vi "Initialize QA Session.vi"(0 "resonator labels":string[](array[string]), 1 "Oximetry Mode?":bool, 5 "Sample Selection":string[](array[string])=["None v1", "T10-1 v1", "T10-10 v1", "T10-11 v1", "T10-12 v1", "T10-13 v1", "T10-14 v1", "T10-15 v1", "T10-16 v1", "T10-17 v1", "T10-2 v1", "T10-3 v1", "T10-4 v1", "T10-5 v1", "T10-6 v1", "T10-7 v1", "T10-8 v1", "T10-9 v1", "T1-10 v1", "T1-11 v1", "T11-1 v1", "T11-10 v1", "T11-11 v1", "T11-12 v1", "T11-13 v1", "T11-14 v1", "T11-15 v1", "T11-16 v1", "T11-17 v1", "T11-18 v1", "T11-19 v1", "T1-12 v1", "T11-2 v1", "T11-20 v1", "T11-21 v1", "T11-22 v1", "T11-23 v1", "T11-24 v1", "T11-25 v1", "T11-26 v1", "T11-27 v1", "T11-28 v1", "T11-29 v1", "T1-13 v1", "T11-3 v1", "T11-30 v1", "T11-31 v1", "T11-32 v1", "T11-33 v1", "T11-34 v1", "T11-35 v1", "T11-36 v1", "T11-37 v1", "T11-38 v1", "T11-39 v1", "T1-14 v1", "T11-4 v1", "T11-40 v1", "T11-41 v1", "T11-42 v1", "T1-15 v1", "T11-5 v1", "T1-16 v1", "T11-6 v1", "T1-17 v1", "T11-7 v1", "T1-18 v1", "T11-8 v1", "T1-19 v1", "T11-9 v1", "T1-2 v1", "T1-2 v2", "T1-2 v3", "T1-20 v1", "T1-21 v1", "T12-1 v1", "T12-10 v1", "T12-11 v1", "T12-12 v1", "T12-13 v1", "T12-14 v1", "T12-15 v1", "T12-16 v1", "T12-17 v1", "T12-18 v1", "T12-19 v1", "T1-22 v1", "T12-2 v1", "T1-23 v1", "T12-3 v1", "T1-24 v1", "T12-4 v1", "T1-25 v1", "T12-5 v1", "T1-26 v1", "T12-6 v1", "T1-27 v1", "T12-7 v1", "T1-28 v1", "T12-8 v1", "T1-29 v1", "T12-9 v1", "T1-3 v1", "T13-10 v1", "T13-11 v1", "T13-12 v1", "T13-13 v1", "T13-2 v1", "T13-3 v1", "T13-4 v1", "T13-5 v1", "T13-6 v1", "T13-7 v1", "T13-8 v1", "T13-9 v1", "T1-4 v1", "T14-1 v1", "T14-10 v1", "T14-11 v1", "T14-12 v1", "T14-13 v1", "T14-14 v1", "T14-15 v1", "T14-16 v1", "T14-17 v1", "T14-2 v1", "T14-3 v1", "T14-4 v1", "T14-5 v1", "T14-6 v1", "T14-7 v1", "T14-8 v1", "T14-9 v1", "T1-5 v1", "T1-5 v2", "T15-1 v1", "T15-10 v1", "T15-11 v1", "T15-2 v1", "T15-3 v1", "T15-4 v1", "T15-5 v1", "T15-6 v1", "T15-7 v1", "T15-8 v1", "T15-9 v1", "T1-6 v1", "T1-6 v2", "T16-1 v1", "T16-10 v1", "T16-11 v1", "T16-12 v1", "T16-13 v1", "T16-14 v1", "T16-15 v1", "T16-16 v1", "T16-17 v1", "T16-18 v1", "T16-19 v1", "T16-2 v1", "T16-20 v1", "T16-21 v1", "T16-22 v1", "T16-23 v1", "T16-24 v1", "T16-25 v1", "T16-3 v1", "T16-4 v1", "T16-5 v1", "T16-6 v1", "T16-7 v1", "T16-8 v1", "T16-9 v1", "T1-7 v1", "T17-1 v1", "T17-10 v1", "T17-11 v1", "T17-12 v1", "T17-13 v1", "T17-14 v1", "T17-15 v1", "T17-16 v1", "T17-17 v1", "T17-2 v1", "T17-3 v1", "T17-4 v1", "T17-5 v1", "T17-6 v1", "T17-7 v1", "T17-8 v1", "T17-9 v1", "T1-8 v1", "T18-1 v1", "T18-2 v1", "T18-3 v1", "T18-4 v1", "T18-5 v1", "T18-6 v1", "T18-7 v1", "T18-8 v1", "T18-9 v1", "T1-9 v1", "T19-1 v1", "T19-10 v1", "T19-11 v1", "T19-12 v1", "T19-13 v1", "T19-14 v1", "T19-15 v1", "T19-16 v1", "T19-17 v1", "T19-18 v1", "T19-19 v1", "T19-2 v1", "T19-3 v1", "T19-4 v1", "T19-5 v1", "T19-6 v1", "T19-7 v1", "T19-8 v1", "T19-9 v1", "T20-1 v1", "T20-10 v1", "T20-11 v1", "T20-12 v1", "T20-13 v1", "T20-14 v1", "T20-2 v1", "T20-3 v1", "T20-4 v1", "T20-5 v1", "T20-6 v1", "T20-7 v1", "T20-8 v1", "T20-9 v1", "T2-1 v1", "T2-10 v1", "T2-11 v1", "T21-1 v1", "T21-10 v1", "T21-11 v1", "T21-12 v1", "T21-13 v1", "T21-14 v1", "T21-15 v1", "T21-16 v1", "T21-17 v1", "T21-18 v1", "T21-19 v1", "T2-12 v1", "T21-20 v1", "T2-13 v1", "T21-3 v1", "T21-4 v1", "T21-5 v1", "T21-6 v1", "T21-7 v1", "T21-8 v1", "T21-9 v1", "T2-2 v1", "T22-1 v1", "T22-10 v1", "T22-11 v1", "T22-12 v1", "T22-13 v1", "T22-14 v1", "T22-15 v1", "T22-16 v1", "T22-17 v1", "T22-18 v1", "T22-19 v1", "T22-2 v1", "T22-3 v1", "T22-4 v1", "T22-5 v1", "T22-6 v1", "T22-7 v1", "T22-8 v1", "T22-9 v1", "T2-3 v1", "T23-1 v1", "T23-10 v1", "T23-11 v1", "T23-12 v1", "T23-13 v1", "T23-14 v1", "T23-15 v1", "T23-16 v1", "T23-17 v1", "T23-18 v1", "T23-19 v1", "T23-2 v1", "T23-20 v1", "T23-21 v1", "T23-22 v1", "T23-23 v1", "T23-24 v1", "T23-25 v1", "T23-3 v1", "T23-4 v1", "T23-5 v1", "T23-6 v1", "T23-7 v1", "T23-8 v1", "T23-9 v1", "T2-4 v1", "T24-1 v1", "T24-10 v1", "T24-11 v1", "T24-12 v1", "T24-13 v1", "T24-14 v1", "T24-2 v1", "T24-3 v1", "T24-4 v1", "T24-5 v1", "T24-6 v1", "T24-7 v1", "T24-8 v1", "T24-9 v1", "T2-5 v1", "T25-1 v1", "T25-10 v1", "T25-11 v1", "T25-12 v1", "T25-13 v1", "T25-14 v1", "T25-15 v1", "T25-16 v1", "T25-17 v1", "T25-18 v1", "T25-19 v1", "T25-2 v1", "T25-20 v1", "T25-21 v1", "T25-22 v1", "T25-23 v1", "T25-24 v1", "T25-25 v1", "T25-26 v1", "T25-27 v1", "T25-3 v1", "T25-4 v1", "T25-5 v1", "T25-6 v1", "T25-7 v1", "T25-8 v1", "T25-9 v1", "T2-6 v1", "T26-1 v1", "T26-10 v1", "T26-11 v1", "T26-12 v1", "T26-13 v1", "T26-14 v1", "T26-15 v1", "T26-16 v1", "T26-17 v1", "T26-18 v1", "T26-19 v1", "T26-2 v1", "T26-20 v1", "T26-21 v1", "T26-22 v1", "T26-23 v1", "T26-24 v1", "T26-25 v1", "T26-26 v1", "T26-3 v1", "T26-4 v1", "T26-5 v1", "T26-6 v1", "T26-7 v1", "T26-8 v1", "T26-9 v1", "T2-7 v1", "T27-1 v1", "T27-10 v1", "T27-11 v1", "T27-12 v1", "T27-13 v1", "T27-14 v1", "T27-15 v1", "T27-16 v1", "T27-17 v1", "T27-18 v1", "T27-19 v1", "T27-2 v1", "T27-20 v1", "T27-21 v1", "T27-22 v1", "T27-23 v1", "T27-24 v1", "T27-25 v1", "T27-3 v1", "T27-4 v1", "T27-5 v1", "T27-6 v1", "T27-7 v1", "T27-8 v1", "T27-9 v1", "T2-8 v1", "T28-1 v1", "T28-2 v1", "T28-3 v1", "T28-4 v1", "T28-5 v1", "T28-6 v1", "T28-7 v1", "T28-8 v1", "T2-9 v1", "T29-1 v1", "T29-10 v1", "T29-11 v1", "T29-12 v1", "T29-13 v1", "T29-14 v1", "T29-15 v1", "T29-16 v1", "T29-17 v1", "T29-18 v1", "T29-19 v1", "T29-2 v1", "T29-20 v1", "T29-3 v1", "T29-4 v1", "T29-5 v1", "T29-6 v1", "T29-7 v1", "T29-8 v1", "T29-9 v1", "T30-1 v1", "T30-10 v1", "T30-11 v1", "T30-12 v1", "T30-13 v1", "T30-14 v1", "T30-15 v1", "T30-16 v1", "T30-17 v1", "T30-18 v1", "T30-19 v1", "T30-2 v1", "T30-3 v1", "T30-4 v1", "T30-5 v1", "T30-6 v1", "T30-7 v1", "T30-8 v1", "T30-9 v1", "T3-1 v1", "T3-10 v1", "T3-11 v1", "T31-1 v1", "T3-12 v1", "T31-2 v1", "T3-13 v1", "T31-3 v1", "T3-14 v1", "T31-4 v1", "T3-15 v1", "T3-16 v1", "T3-2 v1", "T32-1 v1", "T32-10 v1", "T32-11 v1", "T32-12 v1", "T32-13 v1", "T32-14 v1", "T32-15 v1", "T32-16 v1", "T32-17 v1", "T32-18 v1", "T32-19 v1", "T32-2 v1", "T32-3 v1", "T32-4 v1", "T32-5 v1", "T32-6 v1", "T32-7 v1", "T32-8 v1", "T32-9 v1", "T3-3 v1", "T3-4 v1", "T3-5 v1", "T3-6 v1", "T3-7 v1", "T3-8 v1", "T3-9 v1", "T4-1 v1", "T4-10 v1", "T4-2 v1", "T4-3 v1", "T4-4 v1", "T4-5 v1", "T4-6 v1", "T4-7 v1", "T4-8 v1", "T4-9 v1", "T5-1 v1", "T5-10 v1", "T5-11 v1", "T5-12 v1", "T5-13 v1", "T5-14 v1", "T5-15 v1", "T5-16 v1", "T5-17 v1", "T5-18 v1", "T5-19 v1", "T5-2 v1", "T5-3 v1", "T5-4 v1", "T5-5 v1", "T5-6 v1", "T5-7 v1", "T5-8 v1", "T5-9 v1", "T6-1 v1", "T6-10 v1", "T6-11 v1", "T6-12 v1", "T6-13 v1", "T6-14 v1", "T6-15 v1", "T6-16 v1", "T6-17 v1", "T6-18 v1", "T6-19 v1", "T6-2 v1", "T6-20 v1", "T6-21 v1", "T6-22 v1", "T6-3 v1", "T6-4 v1", "T6-5 v1", "T6-6 v1", "T6-7 v1", "T6-8 v1", "T6-9 v1", "T7-1 v1", "T7-10 v1", "T7-11 v1", "T7-12 v1", "T7-13 v1", "T7-14 v1", "T7-15 v1", "T7-16 v1", "T7-17 v1", "T7-2 v1", "T7-3 v1", "T7-4 v1", "T7-5 v1", "T7-6 v1", "T7-7 v1", "T7-8 v1", "T7-9 v1", "T8-1 v1", "T8-10 v1", "T8-11 v1", "T8-12 v1", "T8-13 v1", "T8-14 v1", "T8-15 v1", "T8-16 v1", "T8-17 v1", "T8-18 v1", "T8-19 v1", "T8-2 v1", "T8-20 v1", "T8-21 v1", "T8-22 v1", "T8-23 v1", "T8-23 v2", "T8-24 v1", "T8-25 v1", "T8-26 v1", "T8-27 v1", "T8-28 v1", "T8-29 v1", "T8-3 v1", "T8-30 v1", "T8-31 v1", "T8-32 v1", "T8-33 v1", "T8-34 v1", "T8-35 v1", "T8-6 v1", "T8-7 v1", "T8-8 v1", "T8-9 v1", "T9-1 v1", "T9-10 v1", "T9-11 v1", "T9-12 v1", "T9-13 v1", "T9-14 v1", "T9-15 v1", "T9-16 v1", "T9-17 v1", "T9-18 v1", "T9-19 v1", "T9-2 v1", "T9-20 v1", "T9-21 v1", "T9-22 v1", "T9-23 v1", "T9-24 v1", "T9-3 v1", "T9-4 v1", "T9-5 v1", "T9-6 v1", "T9-7 v1", "T9-8 v1", "T9-9 v1", "V117-9 v1", "V125-9 v1"], 7 "Standard Options":string[](array[string]), 9 "Gases Used":string[](array[string])=["None v1", "T10-1 v1", "T10-10 v1", "T10-11 v1", "T10-12 v1", "T10-13 v1", "T10-14 v1", "T10-15 v1", "T10-16 v1", "T10-17 v1", "T10-2 v1", "T10-3 v1", "T10-4 v1", "T10-5 v1", "T10-6 v1", "T10-7 v1", "T10-8 v1", "T10-9 v1", "T1-10 v1", "T1-11 v1", "T11-1 v1", "T11-10 v1", "T11-11 v1", "T11-12 v1", "T11-13 v1", "T11-14 v1", "T11-15 v1", "T11-16 v1", "T11-17 v1", "T11-18 v1", "T11-19 v1", "T1-12 v1", "T11-2 v1", "T11-20 v1", "T11-21 v1", "T11-22 v1", "T11-23 v1", "T11-24 v1", "T11-25 v1", "T11-26 v1", "T11-27 v1", "T11-28 v1", "T11-29 v1", "T1-13 v1", "T11-3 v1", "T11-30 v1", "T11-31 v1", "T11-32 v1", "T11-33 v1", "T11-34 v1", "T11-35 v1", "T11-36 v1", "T11-37 v1", "T11-38 v1", "T11-39 v1", "T1-14 v1", "T11-4 v1", "T11-40 v1", "T11-41 v1", "T11-42 v1", "T1-15 v1", "T11-5 v1", "T1-16 v1", "T11-6 v1", "T1-17 v1", "T11-7 v1", "T1-18 v1", "T11-8 v1", "T1-19 v1", "T11-9 v1", "T1-2 v1", "T1-2 v2", "T1-2 v3", "T1-20 v1", "T1-21 v1", "T12-1 v1", "T12-10 v1", "T12-11 v1", "T12-12 v1", "T12-13 v1", "T12-14 v1", "T12-15 v1", "T12-16 v1", "T12-17 v1", "T12-18 v1", "T12-19 v1", "T1-22 v1", "T12-2 v1", "T1-23 v1", "T12-3 v1", "T1-24 v1", "T12-4 v1", "T1-25 v1", "T12-5 v1", "T1-26 v1", "T12-6 v1", "T1-27 v1", "T12-7 v1", "T1-28 v1", "T12-8 v1", "T1-29 v1", "T12-9 v1", "T1-3 v1", "T13-10 v1", "T13-11 v1", "T13-12 v1", "T13-13 v1", "T13-2 v1", "T13-3 v1", "T13-4 v1", "T13-5 v1", "T13-6 v1", "T13-7 v1", "T13-8 v1", "T13-9 v1", "T1-4 v1", "T14-1 v1", "T14-10 v1", "T14-11 v1", "T14-12 v1", "T14-13 v1", "T14-14 v1", "T14-15 v1", "T14-16 v1", "T14-17 v1", "T14-2 v1", "T14-3 v1", "T14-4 v1", "T14-5 v1", "T14-6 v1", "T14-7 v1", "T14-8 v1", "T14-9 v1", "T1-5 v1", "T1-5 v2", "T15-1 v1", "T15-10 v1", "T15-11 v1", "T15-2 v1", "T15-3 v1", "T15-4 v1", "T15-5 v1", "T15-6 v1", "T15-7 v1", "T15-8 v1", "T15-9 v1", "T1-6 v1", "T1-6 v2", "T16-1 v1", "T16-10 v1", "T16-11 v1", "T16-12 v1", "T16-13 v1", "T16-14 v1", "T16-15 v1", "T16-16 v1", "T16-17 v1", "T16-18 v1", "T16-19 v1", "T16-2 v1", "T16-20 v1", "T16-21 v1", "T16-22 v1", "T16-23 v1", "T16-24 v1", "T16-25 v1", "T16-3 v1", "T16-4 v1", "T16-5 v1", "T16-6 v1", "T16-7 v1", "T16-8 v1", "T16-9 v1", "T1-7 v1", "T17-1 v1", "T17-10 v1", "T17-11 v1", "T17-12 v1", "T17-13 v1", "T17-14 v1", "T17-15 v1", "T17-16 v1", "T17-17 v1", "T17-2 v1", "T17-3 v1", "T17-4 v1", "T17-5 v1", "T17-6 v1", "T17-7 v1", "T17-8 v1", "T17-9 v1", "T1-8 v1", "T18-1 v1", "T18-2 v1", "T18-3 v1", "T18-4 v1", "T18-5 v1", "T18-6 v1", "T18-7 v1", "T18-8 v1", "T18-9 v1", "T1-9 v1", "T19-1 v1", "T19-10 v1", "T19-11 v1", "T19-12 v1", "T19-13 v1", "T19-14 v1", "T19-15 v1", "T19-16 v1", "T19-17 v1", "T19-18 v1", "T19-19 v1", "T19-2 v1", "T19-3 v1", "T19-4 v1", "T19-5 v1", "T19-6 v1", "T19-7 v1", "T19-8 v1", "T19-9 v1", "T20-1 v1", "T20-10 v1", "T20-11 v1", "T20-12 v1", "T20-13 v1", "T20-14 v1", "T20-2 v1", "T20-3 v1", "T20-4 v1", "T20-5 v1", "T20-6 v1", "T20-7 v1", "T20-8 v1", "T20-9 v1", "T2-1 v1", "T2-10 v1", "T2-11 v1", "T21-1 v1", "T21-10 v1", "T21-11 v1", "T21-12 v1", "T21-13 v1", "T21-14 v1", "T21-15 v1", "T21-16 v1", "T21-17 v1", "T21-18 v1", "T21-19 v1", "T2-12 v1", "T21-20 v1", "T2-13 v1", "T21-3 v1", "T21-4 v1", "T21-5 v1", "T21-6 v1", "T21-7 v1", "T21-8 v1", "T21-9 v1", "T2-2 v1", "T22-1 v1", "T22-10 v1", "T22-11 v1", "T22-12 v1", "T22-13 v1", "T22-14 v1", "T22-15 v1", "T22-16 v1", "T22-17 v1", "T22-18 v1", "T22-19 v1", "T22-2 v1", "T22-3 v1", "T22-4 v1", "T22-5 v1", "T22-6 v1", "T22-7 v1", "T22-8 v1", "T22-9 v1", "T2-3 v1", "T23-1 v1", "T23-10 v1", "T23-11 v1", "T23-12 v1", "T23-13 v1", "T23-14 v1", "T23-15 v1", "T23-16 v1", "T23-17 v1", "T23-18 v1", "T23-19 v1", "T23-2 v1", "T23-20 v1", "T23-21 v1", "T23-22 v1", "T23-23 v1", "T23-24 v1", "T23-25 v1", "T23-3 v1", "T23-4 v1", "T23-5 v1", "T23-6 v1", "T23-7 v1", "T23-8 v1", "T23-9 v1", "T2-4 v1", "T24-1 v1", "T24-10 v1", "T24-11 v1", "T24-12 v1", "T24-13 v1", "T24-14 v1", "T24-2 v1", "T24-3 v1", "T24-4 v1", "T24-5 v1", "T24-6 v1", "T24-7 v1", "T24-8 v1", "T24-9 v1", "T2-5 v1", "T25-1 v1", "T25-10 v1", "T25-11 v1", "T25-12 v1", "T25-13 v1", "T25-14 v1", "T25-15 v1", "T25-16 v1", "T25-17 v1", "T25-18 v1", "T25-19 v1", "T25-2 v1", "T25-20 v1", "T25-21 v1", "T25-22 v1", "T25-23 v1", "T25-24 v1", "T25-25 v1", "T25-26 v1", "T25-27 v1", "T25-3 v1", "T25-4 v1", "T25-5 v1", "T25-6 v1", "T25-7 v1", "T25-8 v1", "T25-9 v1", "T2-6 v1", "T26-1 v1", "T26-10 v1", "T26-11 v1", "T26-12 v1", "T26-13 v1", "T26-14 v1", "T26-15 v1", "T26-16 v1", "T26-17 v1", "T26-18 v1", "T26-19 v1", "T26-2 v1", "T26-20 v1", "T26-21 v1", "T26-22 v1", "T26-23 v1", "T26-24 v1", "T26-25 v1", "T26-26 v1", "T26-3 v1", "T26-4 v1", "T26-5 v1", "T26-6 v1", "T26-7 v1", "T26-8 v1", "T26-9 v1", "T2-7 v1", "T27-1 v1", "T27-10 v1", "T27-11 v1", "T27-12 v1", "T27-13 v1", "T27-14 v1", "T27-15 v1", "T27-16 v1", "T27-17 v1", "T27-18 v1", "T27-19 v1", "T27-2 v1", "T27-20 v1", "T27-21 v1", "T27-22 v1", "T27-23 v1", "T27-24 v1", "T27-25 v1", "T27-3 v1", "T27-4 v1", "T27-5 v1", "T27-6 v1", "T27-7 v1", "T27-8 v1", "T27-9 v1", "T2-8 v1", "T28-1 v1", "T28-2 v1", "T28-3 v1", "T28-4 v1", "T28-5 v1", "T28-6 v1", "T28-7 v1", "T28-8 v1", "T2-9 v1", "T29-1 v1", "T29-10 v1", "T29-11 v1", "T29-12 v1", "T29-13 v1", "T29-14 v1", "T29-15 v1", "T29-16 v1", "T29-17 v1", "T29-18 v1", "T29-19 v1", "T29-2 v1", "T29-20 v1", "T29-3 v1", "T29-4 v1", "T29-5 v1", "T29-6 v1", "T29-7 v1", "T29-8 v1", "T29-9 v1", "T30-1 v1", "T30-10 v1", "T30-11 v1", "T30-12 v1", "T30-13 v1", "T30-14 v1", "T30-15 v1", "T30-16 v1", "T30-17 v1", "T30-18 v1", "T30-19 v1", "T30-2 v1", "T30-3 v1", "T30-4 v1", "T30-5 v1", "T30-6 v1", "T30-7 v1", "T30-8 v1", "T30-9 v1", "T3-1 v1", "T3-10 v1", "T3-11 v1", "T31-1 v1", "T3-12 v1", "T31-2 v1", "T3-13 v1", "T31-3 v1", "T3-14 v1", "T31-4 v1", "T3-15 v1", "T3-16 v1", "T3-2 v1", "T32-1 v1", "T32-10 v1", "T32-11 v1", "T32-12 v1", "T32-13 v1", "T32-14 v1", "T32-15 v1", "T32-16 v1", "T32-17 v1", "T32-18 v1", "T32-19 v1", "T32-2 v1", "T32-3 v1", "T32-4 v1", "T32-5 v1", "T32-6 v1", "T32-7 v1", "T32-8 v1", "T32-9 v1", "T3-3 v1", "T3-4 v1", "T3-5 v1", "T3-6 v1", "T3-7 v1", "T3-8 v1", "T3-9 v1", "T4-1 v1", "T4-10 v1", "T4-2 v1", "T4-3 v1", "T4-4 v1", "T4-5 v1", "T4-6 v1", "T4-7 v1", "T4-8 v1", "T4-9 v1", "T5-1 v1", "T5-10 v1", "T5-11 v1", "T5-12 v1", "T5-13 v1", "T5-14 v1", "T5-15 v1", "T5-16 v1", "T5-17 v1", "T5-18 v1", "T5-19 v1", "T5-2 v1", "T5-3 v1", "T5-4 v1", "T5-5 v1", "T5-6 v1", "T5-7 v1", "T5-8 v1", "T5-9 v1", "T6-1 v1", "T6-10 v1", "T6-11 v1", "T6-12 v1", "T6-13 v1", "T6-14 v1", "T6-15 v1", "T6-16 v1", "T6-17 v1", "T6-18 v1", "T6-19 v1", "T6-2 v1", "T6-20 v1", "T6-21 v1", "T6-22 v1", "T6-3 v1", "T6-4 v1", "T6-5 v1", "T6-6 v1", "T6-7 v1", "T6-8 v1", "T6-9 v1", "T7-1 v1", "T7-10 v1", "T7-11 v1", "T7-12 v1", "T7-13 v1", "T7-14 v1", "T7-15 v1", "T7-16 v1", "T7-17 v1", "T7-2 v1", "T7-3 v1", "T7-4 v1", "T7-5 v1", "T7-6 v1", "T7-7 v1", "T7-8 v1", "T7-9 v1", "T8-1 v1", "T8-10 v1", "T8-11 v1", "T8-12 v1", "T8-13 v1", "T8-14 v1", "T8-15 v1", "T8-16 v1", "T8-17 v1", "T8-18 v1", "T8-19 v1", "T8-2 v1", "T8-20 v1", "T8-21 v1", "T8-22 v1", "T8-23 v1", "T8-23 v2", "T8-24 v1", "T8-25 v1", "T8-26 v1", "T8-27 v1", "T8-28 v1", "T8-29 v1", "T8-3 v1", "T8-30 v1", "T8-31 v1", "T8-32 v1", "T8-33 v1", "T8-34 v1", "T8-35 v1", "T8-6 v1", "T8-7 v1", "T8-8 v1", "T8-9 v1", "T9-1 v1", "T9-10 v1", "T9-11 v1", "T9-12 v1", "T9-13 v1", "T9-14 v1", "T9-15 v1", "T9-16 v1", "T9-17 v1", "T9-18 v1", "T9-19 v1", "T9-2 v1", "T9-20 v1", "T9-21 v1", "T9-22 v1", "T9-23 v1", "T9-24 v1", "T9-3 v1", "T9-4 v1", "T9-5 v1", "T9-6 v1", "T9-7 v1", "T9-8 v1", "T9-9 v1", "V117-9 v1", "V125-9 v1"], 11 "Fraction of Inhaled Oxygen":string[](array[string])=["None v1", "T10-1 v1", "T10-10 v1", "T10-11 v1", "T10-12 v1", "T10-13 v1", "T10-14 v1", "T10-15 v1", "T10-16 v1", "T10-17 v1", "T10-2 v1", "T10-3 v1", "T10-4 v1", "T10-5 v1", "T10-6 v1", "T10-7 v1", "T10-8 v1", "T10-9 v1", "T1-10 v1", "T1-11 v1", "T11-1 v1", "T11-10 v1", "T11-11 v1", "T11-12 v1", "T11-13 v1", "T11-14 v1", "T11-15 v1", "T11-16 v1", "T11-17 v1", "T11-18 v1", "T11-19 v1", "T1-12 v1", "T11-2 v1", "T11-20 v1", "T11-21 v1", "T11-22 v1", "T11-23 v1", "T11-24 v1", "T11-25 v1", "T11-26 v1", "T11-27 v1", "T11-28 v1", "T11-29 v1", "T1-13 v1", "T11-3 v1", "T11-30 v1", "T11-31 v1", "T11-32 v1", "T11-33 v1", "T11-34 v1", "T11-35 v1", "T11-36 v1", "T11-37 v1", "T11-38 v1", "T11-39 v1", "T1-14 v1", "T11-4 v1", "T11-40 v1", "T11-41 v1", "T11-42 v1", "T1-15 v1", "T11-5 v1", "T1-16 v1", "T11-6 v1", "T1-17 v1", "T11-7 v1", "T1-18 v1", "T11-8 v1", "T1-19 v1", "T11-9 v1", "T1-2 v1", "T1-2 v2", "T1-2 v3", "T1-20 v1", "T1-21 v1", "T12-1 v1", "T12-10 v1", "T12-11 v1", "T12-12 v1", "T12-13 v1", "T12-14 v1", "T12-15 v1", "T12-16 v1", "T12-17 v1", "T12-18 v1", "T12-19 v1", "T1-22 v1", "T12-2 v1", "T1-23 v1", "T12-3 v1", "T1-24 v1", "T12-4 v1", "T1-25 v1", "T12-5 v1", "T1-26 v1", "T12-6 v1", "T1-27 v1", "T12-7 v1", "T1-28 v1", "T12-8 v1", "T1-29 v1", "T12-9 v1", "T1-3 v1", "T13-10 v1", "T13-11 v1", "T13-12 v1", "T13-13 v1", "T13-2 v1", "T13-3 v1", "T13-4 v1", "T13-5 v1", "T13-6 v1", "T13-7 v1", "T13-8 v1", "T13-9 v1", "T1-4 v1", "T14-1 v1", "T14-10 v1", "T14-11 v1", "T14-12 v1", "T14-13 v1", "T14-14 v1", "T14-15 v1", "T14-16 v1", "T14-17 v1", "T14-2 v1", "T14-3 v1", "T14-4 v1", "T14-5 v1", "T14-6 v1", "T14-7 v1", "T14-8 v1", "T14-9 v1", "T1-5 v1", "T1-5 v2", "T15-1 v1", "T15-10 v1", "T15-11 v1", "T15-2 v1", "T15-3 v1", "T15-4 v1", "T15-5 v1", "T15-6 v1", "T15-7 v1", "T15-8 v1", "T15-9 v1", "T1-6 v1", "T1-6 v2", "T16-1 v1", "T16-10 v1", "T16-11 v1", "T16-12 v1", "T16-13 v1", "T16-14 v1", "T16-15 v1", "T16-16 v1", "T16-17 v1", "T16-18 v1", "T16-19 v1", "T16-2 v1", "T16-20 v1", "T16-21 v1", "T16-22 v1", "T16-23 v1", "T16-24 v1", "T16-25 v1", "T16-3 v1", "T16-4 v1", "T16-5 v1", "T16-6 v1", "T16-7 v1", "T16-8 v1", "T16-9 v1", "T1-7 v1", "T17-1 v1", "T17-10 v1", "T17-11 v1", "T17-12 v1", "T17-13 v1", "T17-14 v1", "T17-15 v1", "T17-16 v1", "T17-17 v1", "T17-2 v1", "T17-3 v1", "T17-4 v1", "T17-5 v1", "T17-6 v1", "T17-7 v1", "T17-8 v1", "T17-9 v1", "T1-8 v1", "T18-1 v1", "T18-2 v1", "T18-3 v1", "T18-4 v1", "T18-5 v1", "T18-6 v1", "T18-7 v1", "T18-8 v1", "T18-9 v1", "T1-9 v1", "T19-1 v1", "T19-10 v1", "T19-11 v1", "T19-12 v1", "T19-13 v1", "T19-14 v1", "T19-15 v1", "T19-16 v1", "T19-17 v1", "T19-18 v1", "T19-19 v1", "T19-2 v1", "T19-3 v1", "T19-4 v1", "T19-5 v1", "T19-6 v1", "T19-7 v1", "T19-8 v1", "T19-9 v1", "T20-1 v1", "T20-10 v1", "T20-11 v1", "T20-12 v1", "T20-13 v1", "T20-14 v1", "T20-2 v1", "T20-3 v1", "T20-4 v1", "T20-5 v1", "T20-6 v1", "T20-7 v1", "T20-8 v1", "T20-9 v1", "T2-1 v1", "T2-10 v1", "T2-11 v1", "T21-1 v1", "T21-10 v1", "T21-11 v1", "T21-12 v1", "T21-13 v1", "T21-14 v1", "T21-15 v1", "T21-16 v1", "T21-17 v1", "T21-18 v1", "T21-19 v1", "T2-12 v1", "T21-20 v1", "T2-13 v1", "T21-3 v1", "T21-4 v1", "T21-5 v1", "T21-6 v1", "T21-7 v1", "T21-8 v1", "T21-9 v1", "T2-2 v1", "T22-1 v1", "T22-10 v1", "T22-11 v1", "T22-12 v1", "T22-13 v1", "T22-14 v1", "T22-15 v1", "T22-16 v1", "T22-17 v1", "T22-18 v1", "T22-19 v1", "T22-2 v1", "T22-3 v1", "T22-4 v1", "T22-5 v1", "T22-6 v1", "T22-7 v1", "T22-8 v1", "T22-9 v1", "T2-3 v1", "T23-1 v1", "T23-10 v1", "T23-11 v1", "T23-12 v1", "T23-13 v1", "T23-14 v1", "T23-15 v1", "T23-16 v1", "T23-17 v1", "T23-18 v1", "T23-19 v1", "T23-2 v1", "T23-20 v1", "T23-21 v1", "T23-22 v1", "T23-23 v1", "T23-24 v1", "T23-25 v1", "T23-3 v1", "T23-4 v1", "T23-5 v1", "T23-6 v1", "T23-7 v1", "T23-8 v1", "T23-9 v1", "T2-4 v1", "T24-1 v1", "T24-10 v1", "T24-11 v1", "T24-12 v1", "T24-13 v1", "T24-14 v1", "T24-2 v1", "T24-3 v1", "T24-4 v1", "T24-5 v1", "T24-6 v1", "T24-7 v1", "T24-8 v1", "T24-9 v1", "T2-5 v1", "T25-1 v1", "T25-10 v1", "T25-11 v1", "T25-12 v1", "T25-13 v1", "T25-14 v1", "T25-15 v1", "T25-16 v1", "T25-17 v1", "T25-18 v1", "T25-19 v1", "T25-2 v1", "T25-20 v1", "T25-21 v1", "T25-22 v1", "T25-23 v1", "T25-24 v1", "T25-25 v1", "T25-26 v1", "T25-27 v1", "T25-3 v1", "T25-4 v1", "T25-5 v1", "T25-6 v1", "T25-7 v1", "T25-8 v1", "T25-9 v1", "T2-6 v1", "T26-1 v1", "T26-10 v1", "T26-11 v1", "T26-12 v1", "T26-13 v1", "T26-14 v1", "T26-15 v1", "T26-16 v1", "T26-17 v1", "T26-18 v1", "T26-19 v1", "T26-2 v1", "T26-20 v1", "T26-21 v1", "T26-22 v1", "T26-23 v1", "T26-24 v1", "T26-25 v1", "T26-26 v1", "T26-3 v1", "T26-4 v1", "T26-5 v1", "T26-6 v1", "T26-7 v1", "T26-8 v1", "T26-9 v1", "T2-7 v1", "T27-1 v1", "T27-10 v1", "T27-11 v1", "T27-12 v1", "T27-13 v1", "T27-14 v1", "T27-15 v1", "T27-16 v1", "T27-17 v1", "T27-18 v1", "T27-19 v1", "T27-2 v1", "T27-20 v1", "T27-21 v1", "T27-22 v1", "T27-23 v1", "T27-24 v1", "T27-25 v1", "T27-3 v1", "T27-4 v1", "T27-5 v1", "T27-6 v1", "T27-7 v1", "T27-8 v1", "T27-9 v1", "T2-8 v1", "T28-1 v1", "T28-2 v1", "T28-3 v1", "T28-4 v1", "T28-5 v1", "T28-6 v1", "T28-7 v1", "T28-8 v1", "T2-9 v1", "T29-1 v1", "T29-10 v1", "T29-11 v1", "T29-12 v1", "T29-13 v1", "T29-14 v1", "T29-15 v1", "T29-16 v1", "T29-17 v1", "T29-18 v1", "T29-19 v1", "T29-2 v1", "T29-20 v1", "T29-3 v1", "T29-4 v1", "T29-5 v1", "T29-6 v1", "T29-7 v1", "T29-8 v1", "T29-9 v1", "T30-1 v1", "T30-10 v1", "T30-11 v1", "T30-12 v1", "T30-13 v1", "T30-14 v1", "T30-15 v1", "T30-16 v1", "T30-17 v1", "T30-18 v1", "T30-19 v1", "T30-2 v1", "T30-3 v1", "T30-4 v1", "T30-5 v1", "T30-6 v1", "T30-7 v1", "T30-8 v1", "T30-9 v1", "T3-1 v1", "T3-10 v1", "T3-11 v1", "T31-1 v1", "T3-12 v1", "T31-2 v1", "T3-13 v1", "T31-3 v1", "T3-14 v1", "T31-4 v1", "T3-15 v1", "T3-16 v1", "T3-2 v1", "T32-1 v1", "T32-10 v1", "T32-11 v1", "T32-12 v1", "T32-13 v1", "T32-14 v1", "T32-15 v1", "T32-16 v1", "T32-17 v1", "T32-18 v1", "T32-19 v1", "T32-2 v1", "T32-3 v1", "T32-4 v1", "T32-5 v1", "T32-6 v1", "T32-7 v1", "T32-8 v1", "T32-9 v1", "T3-3 v1", "T3-4 v1", "T3-5 v1", "T3-6 v1", "T3-7 v1", "T3-8 v1", "T3-9 v1", "T4-1 v1", "T4-10 v1", "T4-2 v1", "T4-3 v1", "T4-4 v1", "T4-5 v1", "T4-6 v1", "T4-7 v1", "T4-8 v1", "T4-9 v1", "T5-1 v1", "T5-10 v1", "T5-11 v1", "T5-12 v1", "T5-13 v1", "T5-14 v1", "T5-15 v1", "T5-16 v1", "T5-17 v1", "T5-18 v1", "T5-19 v1", "T5-2 v1", "T5-3 v1", "T5-4 v1", "T5-5 v1", "T5-6 v1", "T5-7 v1", "T5-8 v1", "T5-9 v1", "T6-1 v1", "T6-10 v1", "T6-11 v1", "T6-12 v1", "T6-13 v1", "T6-14 v1", "T6-15 v1", "T6-16 v1", "T6-17 v1", "T6-18 v1", "T6-19 v1", "T6-2 v1", "T6-20 v1", "T6-21 v1", "T6-22 v1", "T6-3 v1", "T6-4 v1", "T6-5 v1", "T6-6 v1", "T6-7 v1", "T6-8 v1", "T6-9 v1", "T7-1 v1", "T7-10 v1", "T7-11 v1", "T7-12 v1", "T7-13 v1", "T7-14 v1", "T7-15 v1", "T7-16 v1", "T7-17 v1", "T7-2 v1", "T7-3 v1", "T7-4 v1", "T7-5 v1", "T7-6 v1", "T7-7 v1", "T7-8 v1", "T7-9 v1", "T8-1 v1", "T8-10 v1", "T8-11 v1", "T8-12 v1", "T8-13 v1", "T8-14 v1", "T8-15 v1", "T8-16 v1", "T8-17 v1", "T8-18 v1", "T8-19 v1", "T8-2 v1", "T8-20 v1", "T8-21 v1", "T8-22 v1", "T8-23 v1", "T8-23 v2", "T8-24 v1", "T8-25 v1", "T8-26 v1", "T8-27 v1", "T8-28 v1", "T8-29 v1", "T8-3 v1", "T8-30 v1", "T8-31 v1", "T8-32 v1", "T8-33 v1", "T8-34 v1", "T8-35 v1", "T8-6 v1", "T8-7 v1", "T8-8 v1", "T8-9 v1", "T9-1 v1", "T9-10 v1", "T9-11 v1", "T9-12 v1", "T9-13 v1", "T9-14 v1", "T9-15 v1", "T9-16 v1", "T9-17 v1", "T9-18 v1", "T9-19 v1", "T9-2 v1", "T9-20 v1", "T9-21 v1", "T9-22 v1", "T9-23 v1", "T9-24 v1", "T9-3 v1", "T9-4 v1", "T9-5 v1", "T9-6 v1", "T9-7 v1", "T9-8 v1", "T9-9 v1", "V117-9 v1", "V125-9 v1"], 12 "BallZero Options":string[](array[string]), 13 "IRS Options":string[](array[string])) -> (4 "Resonator ID":string="Inc2", 6 "Sample Selected":string, 10 "Gases Used":string="T10-10 v1", 15 "Sample Type":T1)   [LabVIEW 2016]
uses:
  Types/Sample Type.ctl
panel:
  in  "BallZero Selection":i32(ring)=1
  in  "Standard Tooth Selection":i32(ring)=1
  in  "IRS Selection":i32(ring)=1
  in  "Manual Sample Input":string
  out "Fraction O2":string
  in  "stop":bool
  in  "Fraction of Inhaled Oxygen":i32(ring)=1 items=["None v1", "T10-1 v1", "T10-10 v1", "T10-11 v1", "T10-12 v1", "T10-13 v1", "T10-14 v1", "T10-15 v1", "T10-16 v1", "T10-17 v1", "T10-2 v1", "T10-3 v1", "T10-4 v1", "T10-5 v1", "T10-6 v1", "T10-7 v1", "T10-8 v1", "T10-9 v1", "T1-10 v1", "T1-11 v1", "T11-1 v1", "T11-10 v1", "T11-11 v1", "T11-12 v1", "T11-13 v1", "T11-14 v1", "T11-15 v1", "T11-16 v1", "T11-17 v1", "T11-18 v1", "T11-19 v1", "T1-12 v1", "T11-2 v1", "T11-20 v1", "T11-21 v1", "T11-22 v1", "T11-23 v1", "T11-24 v1", "T11-25 v1", "T11-26 v1", "T11-27 v1", "T11-28 v1", "T11-29 v1", "T1-13 v1", "T11-3 v1", "T11-30 v1", "T11-31 v1", "T11-32 v1", "T11-33 v1", "T11-34 v1", "T11-35 v1", "T11-36 v1", "T11-37 v1", "T11-38 v1", "T11-39 v1", "T1-14 v1", "T11-4 v1", "T11-40 v1", "T11-41 v1", "T11-42 v1", "T1-15 v1", "T11-5 v1", "T1-16 v1", "T11-6 v1", "T1-17 v1", "T11-7 v1", "T1-18 v1", "T11-8 v1", "T1-19 v1", "T11-9 v1", "T1-2 v1", "T1-2 v2", "T1-2 v3", "T1-20 v1", "T1-21 v1", "T12-1 v1", "T12-10 v1", "T12-11 v1", "T12-12 v1", "T12-13 v1", "T12-14 v1", "T12-15 v1", "T12-16 v1", "T12-17 v1", "T12-18 v1", "T12-19 v1", "T1-22 v1", "T12-2 v1", "T1-23 v1", "T12-3 v1", "T1-24 v1", "T12-4 v1", "T1-25 v1", "T12-5 v1", "T1-26 v1", "T12-6 v1", "T1-27 v1", "T12-7 v1", "T1-28 v1", "T12-8 v1", "T1-29 v1", "T12-9 v1", "T1-3 v1", "T13-10 v1", "T13-11 v1", "T13-12 v1", "T13-13 v1", "T13-2 v1", "T13-3 v1", "T13-4 v1", "T13-5 v1", "T13-6 v1", "T13-7 v1", "T13-8 v1", "T13-9 v1", "T1-4 v1", "T14-1 v1", "T14-10 v1", "T14-11 v1", "T14-12 v1", "T14-13 v1", "T14-14 v1", "T14-15 v1", "T14-16 v1", "T14-17 v1", "T14-2 v1", "T14-3 v1", "T14-4 v1", "T14-5 v1", "T14-6 v1", "T14-7 v1", "T14-8 v1", "T14-9 v1", "T1-5 v1", "T1-5 v2", "T15-1 v1", "T15-10 v1", "T15-11 v1", "T15-2 v1", "T15-3 v1", "T15-4 v1", "T15-5 v1", "T15-6 v1", "T15-7 v1", "T15-8 v1", "T15-9 v1", "T1-6 v1", "T1-6 v2", "T16-1 v1", "T16-10 v1", "T16-11 v1", "T16-12 v1", "T16-13 v1", "T16-14 v1", "T16-15 v1", "T16-16 v1", "T16-17 v1", "T16-18 v1", "T16-19 v1", "T16-2 v1", "T16-20 v1", "T16-21 v1", "T16-22 v1", "T16-23 v1", "T16-24 v1", "T16-25 v1", "T16-3 v1", "T16-4 v1", "T16-5 v1", "T16-6 v1", "T16-7 v1", "T16-8 v1", "T16-9 v1", "T1-7 v1", "T17-1 v1", "T17-10 v1", "T17-11 v1", "T17-12 v1", "T17-13 v1", "T17-14 v1", "T17-15 v1", "T17-16 v1", "T17-17 v1", "T17-2 v1", "T17-3 v1", "T17-4 v1", "T17-5 v1", "T17-6 v1", "T17-7 v1", "T17-8 v1", "T17-9 v1", "T1-8 v1", "T18-1 v1", "T18-2 v1", "T18-3 v1", "T18-4 v1", "T18-5 v1", "T18-6 v1", "T18-7 v1", "T18-8 v1", "T18-9 v1", "T1-9 v1", "T19-1 v1", "T19-10 v1", "T19-11 v1", "T19-12 v1", "T19-13 v1", "T19-14 v1", "T19-15 v1", "T19-16 v1", "T19-17 v1", "T19-18 v1", "T19-19 v1", "T19-2 v1", "T19-3 v1", "T19-4 v1", "T19-5 v1", "T19-6 v1", "T19-7 v1", "T19-8 v1", "T19-9 v1", "T20-1 v1", "T20-10 v1", "T20-11 v1", "T20-12 v1", "T20-13 v1", "T20-14 v1", "T20-2 v1", "T20-3 v1", "T20-4 v1", "T20-5 v1", "T20-6 v1", "T20-7 v1", "T20-8 v1", "T20-9 v1", "T2-1 v1", "T2-10 v1", "T2-11 v1", "T21-1 v1", "T21-10 v1", "T21-11 v1", "T21-12 v1", "T21-13 v1", "T21-14 v1", "T21-15 v1", "T21-16 v1", "T21-17 v1", "T21-18 v1", "T21-19 v1", "T2-12 v1", "T21-20 v1", "T2-13 v1", "T21-3 v1", "T21-4 v1", "T21-5 v1", "T21-6 v1", "T21-7 v1", "T21-8 v1", "T21-9 v1", "T2-2 v1", "T22-1 v1", "T22-10 v1", "T22-11 v1", "T22-12 v1", "T22-13 v1", "T22-14 v1", "T22-15 v1", "T22-16 v1", "T22-17 v1", "T22-18 v1", "T22-19 v1", "T22-2 v1", "T22-3 v1", "T22-4 v1", "T22-5 v1", "T22-6 v1", "T22-7 v1", "T22-8 v1", "T22-9 v1", "T2-3 v1", "T23-1 v1", "T23-10 v1", "T23-11 v1", "T23-12 v1", "T23-13 v1", "T23-14 v1", "T23-15 v1", "T23-16 v1", "T23-17 v1", "T23-18 v1", "T23-19 v1", "T23-2 v1", "T23-20 v1", "T23-21 v1", "T23-22 v1", "T23-23 v1", "T23-24 v1", "T23-25 v1", "T23-3 v1", "T23-4 v1", "T23-5 v1", "T23-6 v1", "T23-7 v1", "T23-8 v1", "T23-9 v1", "T2-4 v1", "T24-1 v1", "T24-10 v1", "T24-11 v1", "T24-12 v1", "T24-13 v1", "T24-14 v1", "T24-2 v1", "T24-3 v1", "T24-4 v1", "T24-5 v1", "T24-6 v1", "T24-7 v1", "T24-8 v1", "T24-9 v1", "T2-5 v1", "T25-1 v1", "T25-10 v1", "T25-11 v1", "T25-12 v1", "T25-13 v1", "T25-14 v1", "T25-15 v1", "T25-16 v1", "T25-17 v1", "T25-18 v1", "T25-19 v1", "T25-2 v1", "T25-20 v1", "T25-21 v1", "T25-22 v1", "T25-23 v1", "T25-24 v1", "T25-25 v1", "T25-26 v1", "T25-27 v1", "T25-3 v1", "T25-4 v1", "T25-5 v1", "T25-6 v1", "T25-7 v1", "T25-8 v1", "T25-9 v1", "T2-6 v1", "T26-1 v1", "T26-10 v1", "T26-11 v1", "T26-12 v1", "T26-13 v1", "T26-14 v1", "T26-15 v1", "T26-16 v1", "T26-17 v1", "T26-18 v1", "T26-19 v1", "T26-2 v1", "T26-20 v1", "T26-21 v1", "T26-22 v1", "T26-23 v1", "T26-24 v1", "T26-25 v1", "T26-26 v1", "T26-3 v1", "T26-4 v1", "T26-5 v1", "T26-6 v1", "T26-7 v1", "T26-8 v1", "T26-9 v1", "T2-7 v1", "T27-1 v1", "T27-10 v1", "T27-11 v1", "T27-12 v1", "T27-13 v1", "T27-14 v1", "T27-15 v1", "T27-16 v1", "T27-17 v1", "T27-18 v1", "T27-19 v1", "T27-2 v1", "T27-20 v1", "T27-21 v1", "T27-22 v1", "T27-23 v1", "T27-24 v1", "T27-25 v1", "T27-3 v1", "T27-4 v1", "T27-5 v1", "T27-6 v1", "T27-7 v1", "T27-8 v1", "T27-9 v1", "T2-8 v1", "T28-1 v1", "T28-2 v1", "T28-3 v1", "T28-4 v1", "T28-5 v1", "T28-6 v1", "T28-7 v1", "T28-8 v1", "T2-9 v1", "T29-1 v1", "T29-10 v1", "T29-11 v1", "T29-12 v1", "T29-13 v1", "T29-14 v1", "T29-15 v1", "T29-16 v1", "T29-17 v1", "T29-18 v1", "T29-19 v1", "T29-2 v1", "T29-20 v1", "T29-3 v1", "T29-4 v1", "T29-5 v1", "T29-6 v1", "T29-7 v1", "T29-8 v1", "T29-9 v1", "T30-1 v1", "T30-10 v1", "T30-11 v1", "T30-12 v1", "T30-13 v1", "T30-14 v1", "T30-15 v1", "T30-16 v1", "T30-17 v1", "T30-18 v1", "T30-19 v1", "T30-2 v1", "T30-3 v1", "T30-4 v1", "T30-5 v1", "T30-6 v1", "T30-7 v1", "T30-8 v1", "T30-9 v1", "T3-1 v1", "T3-10 v1", "T3-11 v1", "T31-1 v1", "T3-12 v1", "T31-2 v1", "T3-13 v1", "T31-3 v1", "T3-14 v1", "T31-4 v1", "T3-15 v1", "T3-16 v1", "T3-2 v1", "T32-1 v1", "T32-10 v1", "T32-11 v1", "T32-12 v1", "T32-13 v1", "T32-14 v1", "T32-15 v1", "T32-16 v1", "T32-17 v1", "T32-18 v1", "T32-19 v1", "T32-2 v1", "T32-3 v1", "T32-4 v1", "T32-5 v1", "T32-6 v1", "T32-7 v1", "T32-8 v1", "T32-9 v1", "T3-3 v1", "T3-4 v1", "T3-5 v1", "T3-6 v1", "T3-7 v1", "T3-8 v1", "T3-9 v1", "T4-1 v1", "T4-10 v1", "T4-2 v1", "T4-3 v1", "T4-4 v1", "T4-5 v1", "T4-6 v1", "T4-7 v1", "T4-8 v1", "T4-9 v1", "T5-1 v1", "T5-10 v1", "T5-11 v1", "T5-12 v1", "T5-13 v1", "T5-14 v1", "T5-15 v1", "T5-16 v1", "T5-17 v1", "T5-18 v1", "T5-19 v1", "T5-2 v1", "T5-3 v1", "T5-4 v1", "T5-5 v1", "T5-6 v1", "T5-7 v1", "T5-8 v1", "T5-9 v1", "T6-1 v1", "T6-10 v1", "T6-11 v1", "T6-12 v1", "T6-13 v1", "T6-14 v1", "T6-15 v1", "T6-16 v1", "T6-17 v1", "T6-18 v1", "T6-19 v1", "T6-2 v1", "T6-20 v1", "T6-21 v1", "T6-22 v1", "T6-3 v1", "T6-4 v1", "T6-5 v1", "T6-6 v1", "T6-7 v1", "T6-8 v1", "T6-9 v1", "T7-1 v1", "T7-10 v1", "T7-11 v1", "T7-12 v1", "T7-13 v1", "T7-14 v1", "T7-15 v1", "T7-16 v1", "T7-17 v1", "T7-2 v1", "T7-3 v1", "T7-4 v1", "T7-5 v1", "T7-6 v1", "T7-7 v1", "T7-8 v1", "T7-9 v1", "T8-1 v1", "T8-10 v1", "T8-11 v1", "T8-12 v1", "T8-13 v1", "T8-14 v1", "T8-15 v1", "T8-16 v1", "T8-17 v1", "T8-18 v1", "T8-19 v1", "T8-2 v1", "T8-20 v1", "T8-21 v1", "T8-22 v1", "T8-23 v1", "T8-23 v2", "T8-24 v1", "T8-25 v1", "T8-26 v1", "T8-27 v1", "T8-28 v1", "T8-29 v1", "T8-3 v1", "T8-30 v1", "T8-31 v1", "T8-32 v1", "T8-33 v1", "T8-34 v1", "T8-35 v1", "T8-6 v1", "T8-7 v1", "T8-8 v1", "T8-9 v1", "T9-1 v1", "T9-10 v1", "T9-11 v1", "T9-12 v1", "T9-13 v1", "T9-14 v1", "T9-15 v1", "T9-16 v1", "T9-17 v1", "T9-18 v1", "T9-19 v1", "T9-2 v1", "T9-20 v1", "T9-21 v1", "T9-22 v1", "T9-23 v1", "T9-24 v1", "T9-3 v1", "T9-4 v1", "T9-5 v1", "T9-6 v1", "T9-7 v1", "T9-8 v1", "T9-9 v1", "V117-9 v1", "V125-9 v1"]
  in  "Gases Used":i32(ring)=1 items=["None v1", "T10-1 v1", "T10-10 v1", "T10-11 v1", "T10-12 v1", "T10-13 v1", "T10-14 v1", "T10-15 v1", "T10-16 v1", "T10-17 v1", "T10-2 v1", "T10-3 v1", "T10-4 v1", "T10-5 v1", "T10-6 v1", "T10-7 v1", "T10-8 v1", "T10-9 v1", "T1-10 v1", "T1-11 v1", "T11-1 v1", "T11-10 v1", "T11-11 v1", "T11-12 v1", "T11-13 v1", "T11-14 v1", "T11-15 v1", "T11-16 v1", "T11-17 v1", "T11-18 v1", "T11-19 v1", "T1-12 v1", "T11-2 v1", "T11-20 v1", "T11-21 v1", "T11-22 v1", "T11-23 v1", "T11-24 v1", "T11-25 v1", "T11-26 v1", "T11-27 v1", "T11-28 v1", "T11-29 v1", "T1-13 v1", "T11-3 v1", "T11-30 v1", "T11-31 v1", "T11-32 v1", "T11-33 v1", "T11-34 v1", "T11-35 v1", "T11-36 v1", "T11-37 v1", "T11-38 v1", "T11-39 v1", "T1-14 v1", "T11-4 v1", "T11-40 v1", "T11-41 v1", "T11-42 v1", "T1-15 v1", "T11-5 v1", "T1-16 v1", "T11-6 v1", "T1-17 v1", "T11-7 v1", "T1-18 v1", "T11-8 v1", "T1-19 v1", "T11-9 v1", "T1-2 v1", "T1-2 v2", "T1-2 v3", "T1-20 v1", "T1-21 v1", "T12-1 v1", "T12-10 v1", "T12-11 v1", "T12-12 v1", "T12-13 v1", "T12-14 v1", "T12-15 v1", "T12-16 v1", "T12-17 v1", "T12-18 v1", "T12-19 v1", "T1-22 v1", "T12-2 v1", "T1-23 v1", "T12-3 v1", "T1-24 v1", "T12-4 v1", "T1-25 v1", "T12-5 v1", "T1-26 v1", "T12-6 v1", "T1-27 v1", "T12-7 v1", "T1-28 v1", "T12-8 v1", "T1-29 v1", "T12-9 v1", "T1-3 v1", "T13-10 v1", "T13-11 v1", "T13-12 v1", "T13-13 v1", "T13-2 v1", "T13-3 v1", "T13-4 v1", "T13-5 v1", "T13-6 v1", "T13-7 v1", "T13-8 v1", "T13-9 v1", "T1-4 v1", "T14-1 v1", "T14-10 v1", "T14-11 v1", "T14-12 v1", "T14-13 v1", "T14-14 v1", "T14-15 v1", "T14-16 v1", "T14-17 v1", "T14-2 v1", "T14-3 v1", "T14-4 v1", "T14-5 v1", "T14-6 v1", "T14-7 v1", "T14-8 v1", "T14-9 v1", "T1-5 v1", "T1-5 v2", "T15-1 v1", "T15-10 v1", "T15-11 v1", "T15-2 v1", "T15-3 v1", "T15-4 v1", "T15-5 v1", "T15-6 v1", "T15-7 v1", "T15-8 v1", "T15-9 v1", "T1-6 v1", "T1-6 v2", "T16-1 v1", "T16-10 v1", "T16-11 v1", "T16-12 v1", "T16-13 v1", "T16-14 v1", "T16-15 v1", "T16-16 v1", "T16-17 v1", "T16-18 v1", "T16-19 v1", "T16-2 v1", "T16-20 v1", "T16-21 v1", "T16-22 v1", "T16-23 v1", "T16-24 v1", "T16-25 v1", "T16-3 v1", "T16-4 v1", "T16-5 v1", "T16-6 v1", "T16-7 v1", "T16-8 v1", "T16-9 v1", "T1-7 v1", "T17-1 v1", "T17-10 v1", "T17-11 v1", "T17-12 v1", "T17-13 v1", "T17-14 v1", "T17-15 v1", "T17-16 v1", "T17-17 v1", "T17-2 v1", "T17-3 v1", "T17-4 v1", "T17-5 v1", "T17-6 v1", "T17-7 v1", "T17-8 v1", "T17-9 v1", "T1-8 v1", "T18-1 v1", "T18-2 v1", "T18-3 v1", "T18-4 v1", "T18-5 v1", "T18-6 v1", "T18-7 v1", "T18-8 v1", "T18-9 v1", "T1-9 v1", "T19-1 v1", "T19-10 v1", "T19-11 v1", "T19-12 v1", "T19-13 v1", "T19-14 v1", "T19-15 v1", "T19-16 v1", "T19-17 v1", "T19-18 v1", "T19-19 v1", "T19-2 v1", "T19-3 v1", "T19-4 v1", "T19-5 v1", "T19-6 v1", "T19-7 v1", "T19-8 v1", "T19-9 v1", "T20-1 v1", "T20-10 v1", "T20-11 v1", "T20-12 v1", "T20-13 v1", "T20-14 v1", "T20-2 v1", "T20-3 v1", "T20-4 v1", "T20-5 v1", "T20-6 v1", "T20-7 v1", "T20-8 v1", "T20-9 v1", "T2-1 v1", "T2-10 v1", "T2-11 v1", "T21-1 v1", "T21-10 v1", "T21-11 v1", "T21-12 v1", "T21-13 v1", "T21-14 v1", "T21-15 v1", "T21-16 v1", "T21-17 v1", "T21-18 v1", "T21-19 v1", "T2-12 v1", "T21-20 v1", "T2-13 v1", "T21-3 v1", "T21-4 v1", "T21-5 v1", "T21-6 v1", "T21-7 v1", "T21-8 v1", "T21-9 v1", "T2-2 v1", "T22-1 v1", "T22-10 v1", "T22-11 v1", "T22-12 v1", "T22-13 v1", "T22-14 v1", "T22-15 v1", "T22-16 v1", "T22-17 v1", "T22-18 v1", "T22-19 v1", "T22-2 v1", "T22-3 v1", "T22-4 v1", "T22-5 v1", "T22-6 v1", "T22-7 v1", "T22-8 v1", "T22-9 v1", "T2-3 v1", "T23-1 v1", "T23-10 v1", "T23-11 v1", "T23-12 v1", "T23-13 v1", "T23-14 v1", "T23-15 v1", "T23-16 v1", "T23-17 v1", "T23-18 v1", "T23-19 v1", "T23-2 v1", "T23-20 v1", "T23-21 v1", "T23-22 v1", "T23-23 v1", "T23-24 v1", "T23-25 v1", "T23-3 v1", "T23-4 v1", "T23-5 v1", "T23-6 v1", "T23-7 v1", "T23-8 v1", "T23-9 v1", "T2-4 v1", "T24-1 v1", "T24-10 v1", "T24-11 v1", "T24-12 v1", "T24-13 v1", "T24-14 v1", "T24-2 v1", "T24-3 v1", "T24-4 v1", "T24-5 v1", "T24-6 v1", "T24-7 v1", "T24-8 v1", "T24-9 v1", "T2-5 v1", "T25-1 v1", "T25-10 v1", "T25-11 v1", "T25-12 v1", "T25-13 v1", "T25-14 v1", "T25-15 v1", "T25-16 v1", "T25-17 v1", "T25-18 v1", "T25-19 v1", "T25-2 v1", "T25-20 v1", "T25-21 v1", "T25-22 v1", "T25-23 v1", "T25-24 v1", "T25-25 v1", "T25-26 v1", "T25-27 v1", "T25-3 v1", "T25-4 v1", "T25-5 v1", "T25-6 v1", "T25-7 v1", "T25-8 v1", "T25-9 v1", "T2-6 v1", "T26-1 v1", "T26-10 v1", "T26-11 v1", "T26-12 v1", "T26-13 v1", "T26-14 v1", "T26-15 v1", "T26-16 v1", "T26-17 v1", "T26-18 v1", "T26-19 v1", "T26-2 v1", "T26-20 v1", "T26-21 v1", "T26-22 v1", "T26-23 v1", "T26-24 v1", "T26-25 v1", "T26-26 v1", "T26-3 v1", "T26-4 v1", "T26-5 v1", "T26-6 v1", "T26-7 v1", "T26-8 v1", "T26-9 v1", "T2-7 v1", "T27-1 v1", "T27-10 v1", "T27-11 v1", "T27-12 v1", "T27-13 v1", "T27-14 v1", "T27-15 v1", "T27-16 v1", "T27-17 v1", "T27-18 v1", "T27-19 v1", "T27-2 v1", "T27-20 v1", "T27-21 v1", "T27-22 v1", "T27-23 v1", "T27-24 v1", "T27-25 v1", "T27-3 v1", "T27-4 v1", "T27-5 v1", "T27-6 v1", "T27-7 v1", "T27-8 v1", "T27-9 v1", "T2-8 v1", "T28-1 v1", "T28-2 v1", "T28-3 v1", "T28-4 v1", "T28-5 v1", "T28-6 v1", "T28-7 v1", "T28-8 v1", "T2-9 v1", "T29-1 v1", "T29-10 v1", "T29-11 v1", "T29-12 v1", "T29-13 v1", "T29-14 v1", "T29-15 v1", "T29-16 v1", "T29-17 v1", "T29-18 v1", "T29-19 v1", "T29-2 v1", "T29-20 v1", "T29-3 v1", "T29-4 v1", "T29-5 v1", "T29-6 v1", "T29-7 v1", "T29-8 v1", "T29-9 v1", "T30-1 v1", "T30-10 v1", "T30-11 v1", "T30-12 v1", "T30-13 v1", "T30-14 v1", "T30-15 v1", "T30-16 v1", "T30-17 v1", "T30-18 v1", "T30-19 v1", "T30-2 v1", "T30-3 v1", "T30-4 v1", "T30-5 v1", "T30-6 v1", "T30-7 v1", "T30-8 v1", "T30-9 v1", "T3-1 v1", "T3-10 v1", "T3-11 v1", "T31-1 v1", "T3-12 v1", "T31-2 v1", "T3-13 v1", "T31-3 v1", "T3-14 v1", "T31-4 v1", "T3-15 v1", "T3-16 v1", "T3-2 v1", "T32-1 v1", "T32-10 v1", "T32-11 v1", "T32-12 v1", "T32-13 v1", "T32-14 v1", "T32-15 v1", "T32-16 v1", "T32-17 v1", "T32-18 v1", "T32-19 v1", "T32-2 v1", "T32-3 v1", "T32-4 v1", "T32-5 v1", "T32-6 v1", "T32-7 v1", "T32-8 v1", "T32-9 v1", "T3-3 v1", "T3-4 v1", "T3-5 v1", "T3-6 v1", "T3-7 v1", "T3-8 v1", "T3-9 v1", "T4-1 v1", "T4-10 v1", "T4-2 v1", "T4-3 v1", "T4-4 v1", "T4-5 v1", "T4-6 v1", "T4-7 v1", "T4-8 v1", "T4-9 v1", "T5-1 v1", "T5-10 v1", "T5-11 v1", "T5-12 v1", "T5-13 v1", "T5-14 v1", "T5-15 v1", "T5-16 v1", "T5-17 v1", "T5-18 v1", "T5-19 v1", "T5-2 v1", "T5-3 v1", "T5-4 v1", "T5-5 v1", "T5-6 v1", "T5-7 v1", "T5-8 v1", "T5-9 v1", "T6-1 v1", "T6-10 v1", "T6-11 v1", "T6-12 v1", "T6-13 v1", "T6-14 v1", "T6-15 v1", "T6-16 v1", "T6-17 v1", "T6-18 v1", "T6-19 v1", "T6-2 v1", "T6-20 v1", "T6-21 v1", "T6-22 v1", "T6-3 v1", "T6-4 v1", "T6-5 v1", "T6-6 v1", "T6-7 v1", "T6-8 v1", "T6-9 v1", "T7-1 v1", "T7-10 v1", "T7-11 v1", "T7-12 v1", "T7-13 v1", "T7-14 v1", "T7-15 v1", "T7-16 v1", "T7-17 v1", "T7-2 v1", "T7-3 v1", "T7-4 v1", "T7-5 v1", "T7-6 v1", "T7-7 v1", "T7-8 v1", "T7-9 v1", "T8-1 v1", "T8-10 v1", "T8-11 v1", "T8-12 v1", "T8-13 v1", "T8-14 v1", "T8-15 v1", "T8-16 v1", "T8-17 v1", "T8-18 v1", "T8-19 v1", "T8-2 v1", "T8-20 v1", "T8-21 v1", "T8-22 v1", "T8-23 v1", "T8-23 v2", "T8-24 v1", "T8-25 v1", "T8-26 v1", "T8-27 v1", "T8-28 v1", "T8-29 v1", "T8-3 v1", "T8-30 v1", "T8-31 v1", "T8-32 v1", "T8-33 v1", "T8-34 v1", "T8-35 v1", "T8-6 v1", "T8-7 v1", "T8-8 v1", "T8-9 v1", "T9-1 v1", "T9-10 v1", "T9-11 v1", "T9-12 v1", "T9-13 v1", "T9-14 v1", "T9-15 v1", "T9-16 v1", "T9-17 v1", "T9-18 v1", "T9-19 v1", "T9-2 v1", "T9-20 v1", "T9-21 v1", "T9-22 v1", "T9-23 v1", "T9-24 v1", "T9-3 v1", "T9-4 v1", "T9-5 v1", "T9-6 v1", "T9-7 v1", "T9-8 v1", "T9-9 v1", "V117-9 v1", "V125-9 v1"]
  in  "Sample Selection":i32(ring)=1 items=["None v1", "T10-1 v1", "T10-10 v1", "T10-11 v1", "T10-12 v1", "T10-13 v1", "T10-14 v1", "T10-15 v1", "T10-16 v1", "T10-17 v1", "T10-2 v1", "T10-3 v1", "T10-4 v1", "T10-5 v1", "T10-6 v1", "T10-7 v1", "T10-8 v1", "T10-9 v1", "T1-10 v1", "T1-11 v1", "T11-1 v1", "T11-10 v1", "T11-11 v1", "T11-12 v1", "T11-13 v1", "T11-14 v1", "T11-15 v1", "T11-16 v1", "T11-17 v1", "T11-18 v1", "T11-19 v1", "T1-12 v1", "T11-2 v1", "T11-20 v1", "T11-21 v1", "T11-22 v1", "T11-23 v1", "T11-24 v1", "T11-25 v1", "T11-26 v1", "T11-27 v1", "T11-28 v1", "T11-29 v1", "T1-13 v1", "T11-3 v1", "T11-30 v1", "T11-31 v1", "T11-32 v1", "T11-33 v1", "T11-34 v1", "T11-35 v1", "T11-36 v1", "T11-37 v1", "T11-38 v1", "T11-39 v1", "T1-14 v1", "T11-4 v1", "T11-40 v1", "T11-41 v1", "T11-42 v1", "T1-15 v1", "T11-5 v1", "T1-16 v1", "T11-6 v1", "T1-17 v1", "T11-7 v1", "T1-18 v1", "T11-8 v1", "T1-19 v1", "T11-9 v1", "T1-2 v1", "T1-2 v2", "T1-2 v3", "T1-20 v1", "T1-21 v1", "T12-1 v1", "T12-10 v1", "T12-11 v1", "T12-12 v1", "T12-13 v1", "T12-14 v1", "T12-15 v1", "T12-16 v1", "T12-17 v1", "T12-18 v1", "T12-19 v1", "T1-22 v1", "T12-2 v1", "T1-23 v1", "T12-3 v1", "T1-24 v1", "T12-4 v1", "T1-25 v1", "T12-5 v1", "T1-26 v1", "T12-6 v1", "T1-27 v1", "T12-7 v1", "T1-28 v1", "T12-8 v1", "T1-29 v1", "T12-9 v1", "T1-3 v1", "T13-10 v1", "T13-11 v1", "T13-12 v1", "T13-13 v1", "T13-2 v1", "T13-3 v1", "T13-4 v1", "T13-5 v1", "T13-6 v1", "T13-7 v1", "T13-8 v1", "T13-9 v1", "T1-4 v1", "T14-1 v1", "T14-10 v1", "T14-11 v1", "T14-12 v1", "T14-13 v1", "T14-14 v1", "T14-15 v1", "T14-16 v1", "T14-17 v1", "T14-2 v1", "T14-3 v1", "T14-4 v1", "T14-5 v1", "T14-6 v1", "T14-7 v1", "T14-8 v1", "T14-9 v1", "T1-5 v1", "T1-5 v2", "T15-1 v1", "T15-10 v1", "T15-11 v1", "T15-2 v1", "T15-3 v1", "T15-4 v1", "T15-5 v1", "T15-6 v1", "T15-7 v1", "T15-8 v1", "T15-9 v1", "T1-6 v1", "T1-6 v2", "T16-1 v1", "T16-10 v1", "T16-11 v1", "T16-12 v1", "T16-13 v1", "T16-14 v1", "T16-15 v1", "T16-16 v1", "T16-17 v1", "T16-18 v1", "T16-19 v1", "T16-2 v1", "T16-20 v1", "T16-21 v1", "T16-22 v1", "T16-23 v1", "T16-24 v1", "T16-25 v1", "T16-3 v1", "T16-4 v1", "T16-5 v1", "T16-6 v1", "T16-7 v1", "T16-8 v1", "T16-9 v1", "T1-7 v1", "T17-1 v1", "T17-10 v1", "T17-11 v1", "T17-12 v1", "T17-13 v1", "T17-14 v1", "T17-15 v1", "T17-16 v1", "T17-17 v1", "T17-2 v1", "T17-3 v1", "T17-4 v1", "T17-5 v1", "T17-6 v1", "T17-7 v1", "T17-8 v1", "T17-9 v1", "T1-8 v1", "T18-1 v1", "T18-2 v1", "T18-3 v1", "T18-4 v1", "T18-5 v1", "T18-6 v1", "T18-7 v1", "T18-8 v1", "T18-9 v1", "T1-9 v1", "T19-1 v1", "T19-10 v1", "T19-11 v1", "T19-12 v1", "T19-13 v1", "T19-14 v1", "T19-15 v1", "T19-16 v1", "T19-17 v1", "T19-18 v1", "T19-19 v1", "T19-2 v1", "T19-3 v1", "T19-4 v1", "T19-5 v1", "T19-6 v1", "T19-7 v1", "T19-8 v1", "T19-9 v1", "T20-1 v1", "T20-10 v1", "T20-11 v1", "T20-12 v1", "T20-13 v1", "T20-14 v1", "T20-2 v1", "T20-3 v1", "T20-4 v1", "T20-5 v1", "T20-6 v1", "T20-7 v1", "T20-8 v1", "T20-9 v1", "T2-1 v1", "T2-10 v1", "T2-11 v1", "T21-1 v1", "T21-10 v1", "T21-11 v1", "T21-12 v1", "T21-13 v1", "T21-14 v1", "T21-15 v1", "T21-16 v1", "T21-17 v1", "T21-18 v1", "T21-19 v1", "T2-12 v1", "T21-20 v1", "T2-13 v1", "T21-3 v1", "T21-4 v1", "T21-5 v1", "T21-6 v1", "T21-7 v1", "T21-8 v1", "T21-9 v1", "T2-2 v1", "T22-1 v1", "T22-10 v1", "T22-11 v1", "T22-12 v1", "T22-13 v1", "T22-14 v1", "T22-15 v1", "T22-16 v1", "T22-17 v1", "T22-18 v1", "T22-19 v1", "T22-2 v1", "T22-3 v1", "T22-4 v1", "T22-5 v1", "T22-6 v1", "T22-7 v1", "T22-8 v1", "T22-9 v1", "T2-3 v1", "T23-1 v1", "T23-10 v1", "T23-11 v1", "T23-12 v1", "T23-13 v1", "T23-14 v1", "T23-15 v1", "T23-16 v1", "T23-17 v1", "T23-18 v1", "T23-19 v1", "T23-2 v1", "T23-20 v1", "T23-21 v1", "T23-22 v1", "T23-23 v1", "T23-24 v1", "T23-25 v1", "T23-3 v1", "T23-4 v1", "T23-5 v1", "T23-6 v1", "T23-7 v1", "T23-8 v1", "T23-9 v1", "T2-4 v1", "T24-1 v1", "T24-10 v1", "T24-11 v1", "T24-12 v1", "T24-13 v1", "T24-14 v1", "T24-2 v1", "T24-3 v1", "T24-4 v1", "T24-5 v1", "T24-6 v1", "T24-7 v1", "T24-8 v1", "T24-9 v1", "T2-5 v1", "T25-1 v1", "T25-10 v1", "T25-11 v1", "T25-12 v1", "T25-13 v1", "T25-14 v1", "T25-15 v1", "T25-16 v1", "T25-17 v1", "T25-18 v1", "T25-19 v1", "T25-2 v1", "T25-20 v1", "T25-21 v1", "T25-22 v1", "T25-23 v1", "T25-24 v1", "T25-25 v1", "T25-26 v1", "T25-27 v1", "T25-3 v1", "T25-4 v1", "T25-5 v1", "T25-6 v1", "T25-7 v1", "T25-8 v1", "T25-9 v1", "T2-6 v1", "T26-1 v1", "T26-10 v1", "T26-11 v1", "T26-12 v1", "T26-13 v1", "T26-14 v1", "T26-15 v1", "T26-16 v1", "T26-17 v1", "T26-18 v1", "T26-19 v1", "T26-2 v1", "T26-20 v1", "T26-21 v1", "T26-22 v1", "T26-23 v1", "T26-24 v1", "T26-25 v1", "T26-26 v1", "T26-3 v1", "T26-4 v1", "T26-5 v1", "T26-6 v1", "T26-7 v1", "T26-8 v1", "T26-9 v1", "T2-7 v1", "T27-1 v1", "T27-10 v1", "T27-11 v1", "T27-12 v1", "T27-13 v1", "T27-14 v1", "T27-15 v1", "T27-16 v1", "T27-17 v1", "T27-18 v1", "T27-19 v1", "T27-2 v1", "T27-20 v1", "T27-21 v1", "T27-22 v1", "T27-23 v1", "T27-24 v1", "T27-25 v1", "T27-3 v1", "T27-4 v1", "T27-5 v1", "T27-6 v1", "T27-7 v1", "T27-8 v1", "T27-9 v1", "T2-8 v1", "T28-1 v1", "T28-2 v1", "T28-3 v1", "T28-4 v1", "T28-5 v1", "T28-6 v1", "T28-7 v1", "T28-8 v1", "T2-9 v1", "T29-1 v1", "T29-10 v1", "T29-11 v1", "T29-12 v1", "T29-13 v1", "T29-14 v1", "T29-15 v1", "T29-16 v1", "T29-17 v1", "T29-18 v1", "T29-19 v1", "T29-2 v1", "T29-20 v1", "T29-3 v1", "T29-4 v1", "T29-5 v1", "T29-6 v1", "T29-7 v1", "T29-8 v1", "T29-9 v1", "T30-1 v1", "T30-10 v1", "T30-11 v1", "T30-12 v1", "T30-13 v1", "T30-14 v1", "T30-15 v1", "T30-16 v1", "T30-17 v1", "T30-18 v1", "T30-19 v1", "T30-2 v1", "T30-3 v1", "T30-4 v1", "T30-5 v1", "T30-6 v1", "T30-7 v1", "T30-8 v1", "T30-9 v1", "T3-1 v1", "T3-10 v1", "T3-11 v1", "T31-1 v1", "T3-12 v1", "T31-2 v1", "T3-13 v1", "T31-3 v1", "T3-14 v1", "T31-4 v1", "T3-15 v1", "T3-16 v1", "T3-2 v1", "T32-1 v1", "T32-10 v1", "T32-11 v1", "T32-12 v1", "T32-13 v1", "T32-14 v1", "T32-15 v1", "T32-16 v1", "T32-17 v1", "T32-18 v1", "T32-19 v1", "T32-2 v1", "T32-3 v1", "T32-4 v1", "T32-5 v1", "T32-6 v1", "T32-7 v1", "T32-8 v1", "T32-9 v1", "T3-3 v1", "T3-4 v1", "T3-5 v1", "T3-6 v1", "T3-7 v1", "T3-8 v1", "T3-9 v1", "T4-1 v1", "T4-10 v1", "T4-2 v1", "T4-3 v1", "T4-4 v1", "T4-5 v1", "T4-6 v1", "T4-7 v1", "T4-8 v1", "T4-9 v1", "T5-1 v1", "T5-10 v1", "T5-11 v1", "T5-12 v1", "T5-13 v1", "T5-14 v1", "T5-15 v1", "T5-16 v1", "T5-17 v1", "T5-18 v1", "T5-19 v1", "T5-2 v1", "T5-3 v1", "T5-4 v1", "T5-5 v1", "T5-6 v1", "T5-7 v1", "T5-8 v1", "T5-9 v1", "T6-1 v1", "T6-10 v1", "T6-11 v1", "T6-12 v1", "T6-13 v1", "T6-14 v1", "T6-15 v1", "T6-16 v1", "T6-17 v1", "T6-18 v1", "T6-19 v1", "T6-2 v1", "T6-20 v1", "T6-21 v1", "T6-22 v1", "T6-3 v1", "T6-4 v1", "T6-5 v1", "T6-6 v1", "T6-7 v1", "T6-8 v1", "T6-9 v1", "T7-1 v1", "T7-10 v1", "T7-11 v1", "T7-12 v1", "T7-13 v1", "T7-14 v1", "T7-15 v1", "T7-16 v1", "T7-17 v1", "T7-2 v1", "T7-3 v1", "T7-4 v1", "T7-5 v1", "T7-6 v1", "T7-7 v1", "T7-8 v1", "T7-9 v1", "T8-1 v1", "T8-10 v1", "T8-11 v1", "T8-12 v1", "T8-13 v1", "T8-14 v1", "T8-15 v1", "T8-16 v1", "T8-17 v1", "T8-18 v1", "T8-19 v1", "T8-2 v1", "T8-20 v1", "T8-21 v1", "T8-22 v1", "T8-23 v1", "T8-23 v2", "T8-24 v1", "T8-25 v1", "T8-26 v1", "T8-27 v1", "T8-28 v1", "T8-29 v1", "T8-3 v1", "T8-30 v1", "T8-31 v1", "T8-32 v1", "T8-33 v1", "T8-34 v1", "T8-35 v1", "T8-6 v1", "T8-7 v1", "T8-8 v1", "T8-9 v1", "T9-1 v1", "T9-10 v1", "T9-11 v1", "T9-12 v1", "T9-13 v1", "T9-14 v1", "T9-15 v1", "T9-16 v1", "T9-17 v1", "T9-18 v1", "T9-19 v1", "T9-2 v1", "T9-20 v1", "T9-21 v1", "T9-22 v1", "T9-23 v1", "T9-24 v1", "T9-3 v1", "T9-4 v1", "T9-5 v1", "T9-6 v1", "T9-7 v1", "T9-8 v1", "T9-9 v1", "V117-9 v1", "V125-9 v1"]
  in  "Resonator":i32(ring)
  # "EPR Input Parameters"
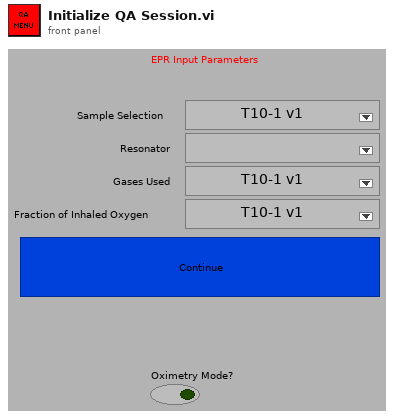
[diagram p1: front panel]
types:
  T1 = typedef "Sample Type.ctl" = enum16{"Empty Resonator", "IRS", "BallZero", "Irradiated Tooth", "Non-irradiated Tooth", "OxyChip", "LiPc", "PDT", "India Ink"}
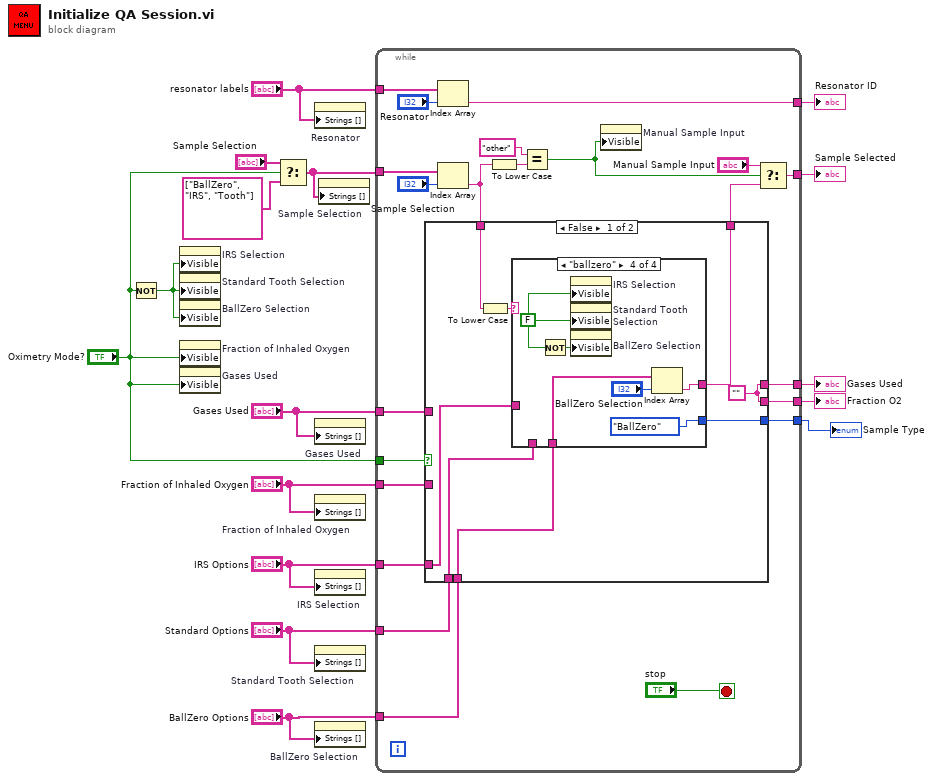
[diagram p0: block diagram]
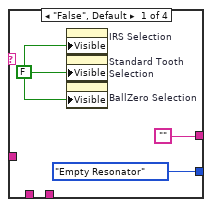
[diagram p2: hidden frame]
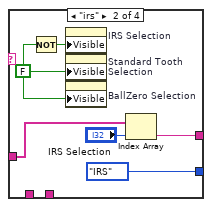
[diagram p3: hidden frame]
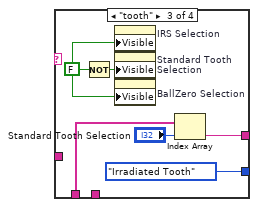
[diagram p4: hidden frame]
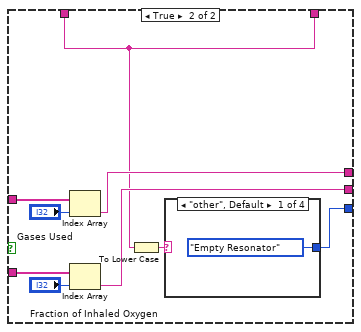
[diagram p5: hidden frame]
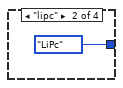
[diagram p6: hidden frame]
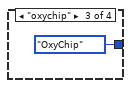
[diagram p7: hidden frame]
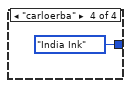
[diagram p8: hidden frame]
diagram:
  n1 = Not(x="Oximetry Mode?") -> (.not. x?=w9:bool)
  n2 = property on="IRS Selection" class="Ring (strict)"("Visible"=w9) -> ()  [unwired: 2 in, 2 out]
  n3 = property on="Standard Tooth Selection" class="Ring (strict)"("Visible"=w9) -> ()  [unwired: 2 in, 2 out]
  n4 = property on="BallZero Selection" class="Ring (strict)"("Visible"=w9) -> ()  [unwired: 2 in, 2 out]
  n5 = property on="Fraction of Inhaled Oxygen" class="Ring (strict)"("Visible"="Oximetry Mode?") -> ()  [unwired: 2 in, 2 out]
  n6 = property on="Gases Used" class="Ring (strict)"("Visible"="Oximetry Mode?") -> ()  [unwired: 2 in, 2 out]
  n7 = Select(t="Sample Selection", s="Oximetry Mode?", f=string[] ["BallZero", "IRS", "Tooth"]) -> (s? t:f=w3:string[])
  n8 = property on="Resonator" class="Ring (strict)"("Strings []"="resonator labels") -> ()  [unwired: 2 in, 2 out]
  n9 = property on="Gases Used" class="Ring (strict)"("Strings []"="Gases Used") -> ()  [unwired: 2 in, 2 out]
  n10 = property on="Fraction of Inhaled Oxygen" class="Ring (strict)"("Strings []"="Fraction of Inhaled Oxygen") -> ()  [unwired: 2 in, 2 out]
  n11 = property on="IRS Selection" class="Ring (strict)"("Strings []"="IRS Options") -> ()  [unwired: 2 in, 2 out]
  n12 = property on="Standard Tooth Selection" class="Ring (strict)"("Strings []"="Standard Options") -> ()  [unwired: 2 in, 2 out]
  n13 = property on="BallZero Selection" class="Ring (strict)"("Strings []"="BallZero Options") -> ()  [unwired: 2 in, 2 out]
  n14 = property on="Sample Selection" class="Ring (strict)"("Strings []"=w3) -> ()  [unwired: 2 in, 2 out]
  n15 = while {
    tunnel: w3 -> [w38]
    tunnel: "resonator labels" -> [w37]
    tunnel: "Gases Used" -> [w32]
    tunnel: "Fraction of Inhaled Oxygen" -> [w30]
    tunnel: [w33] -> w13
    tunnel: [w26] -> w12
    tunnel: [w31] -> w11
    tunnel: [w29] -> w10
    tunnel: "IRS Options" -> [w22]
    tunnel: "Standard Options" -> [w21]
    tunnel: "BallZero Options" -> [w20]
    tunnel: "Oximetry Mode?" -> [w23]
    tunnel: [w17] -> w1
    stop <- "stop" stop-if-true
    n16 = Index Array(array=w37, index="Resonator") -> (element=w33:string)
    n17 = Index Array(array=w38, index="Sample Selection") -> (element=w19:string)
    n18 = case shown="False" w23 {
      tunnel: w32 -> [_ w75]
      tunnel: [w46 w74] -> w31
      tunnel: w30 -> [_ w72]
      tunnel: [w46 w71] -> w29
      tunnel: w22 -> [w43 _]
      tunnel: w21 -> [w41 _]
      tunnel: w20 -> [w40 _]
      tunnel: w19 -> [w45 w69]
      tunnel: [w42 w69] -> w18
      tunnel: [w39 w70] -> w17
      frame False {
        w46 = ""
        n19 = To Lower Case(string=w45) -> (all lower case string=w44:string)
        n20 = case shown="\"ballzero\"" w44 {
          tunnel: w43 -> [_ w52 _ _]
          tunnel: ["" w51 w57 w63] -> w42
          tunnel: w41 -> [_ _ w58 _]
          tunnel: w40 -> [_ _ _ w64]
          tunnel: [Sample_Type."Empty Resonator" ("Sample Type") Sample_Type."IRS" ("Sample Type") Sample_Type."Irradiated Tooth" ("Sample Type") Sample_Type."BallZero" ("Sample Type")] -> w39
          frame "False", Default {
            w49 = FALSE ("Visible")
            n21 = property on="IRS Selection" class="Ring (strict)"("Visible"=w49) -> ()  [unwired: 2 in, 2 out]
            n22 = property on="Standard Tooth Selection" class="Ring (strict)"("Visible"=w49) -> ()  [unwired: 2 in, 2 out]
            n23 = property on="BallZero Selection" class="Ring (strict)"("Visible"=w49) -> ()  [unwired: 2 in, 2 out]
          }
          frame "irs" {
            w54 = FALSE ("Visible")
            n24 = Not(x=w54) -> (.not. x?=w55:bool)
            n25 = property on="IRS Selection" class="Ring (strict)"("Visible"=w55) -> ()  [unwired: 2 in, 2 out]
            n26 = property on="Standard Tooth Selection" class="Ring (strict)"("Visible"=w54) -> ()  [unwired: 2 in, 2 out]
            n27 = property on="BallZero Selection" class="Ring (strict)"("Visible"=w54) -> ()  [unwired: 2 in, 2 out]
            n28 = Index Array(array=w52, index="IRS Selection") -> (element=w51:string)
          }
          frame "tooth" {
            w60 = FALSE ("Visible")
            n29 = Not(x=w60) -> (.not. x?=w61:bool)
            n30 = property on="IRS Selection" class="Ring (strict)"("Visible"=w60) -> ()  [unwired: 2 in, 2 out]
            n31 = property on="Standard Tooth Selection" class="Ring (strict)"("Visible"=w61) -> ()  [unwired: 2 in, 2 out]
            n32 = property on="BallZero Selection" class="Ring (strict)"("Visible"=w60) -> ()  [unwired: 2 in, 2 out]
            n33 = Index Array(array=w58, index="Standard Tooth Selection") -> (element=w57:string)
          }
          frame "ballzero" {
            w66 = FALSE ("Visible")
            n34 = Not(x=w66) -> (.not. x?=w67:bool)
            n35 = property on="IRS Selection" class="Ring (strict)"("Visible"=w66) -> ()  [unwired: 2 in, 2 out]
            n36 = property on="Standard Tooth Selection" class="Ring (strict)"("Visible"=w66) -> ()  [unwired: 2 in, 2 out]
            n37 = property on="BallZero Selection" class="Ring (strict)"("Visible"=w67) -> ()  [unwired: 2 in, 2 out]
            n38 = Index Array(array=w64, index="BallZero Selection") -> (element=w63:string)
          }
        }
      }
      frame True {
        n39 = Index Array(array=w75, index="Gases Used") -> (element=w74:string)
        n40 = Index Array(array=w72, index="Fraction of Inhaled Oxygen") -> (element=w71:string)
        n41 = To Lower Case(string=w69) -> (all lower case string=w68:string)
        n42 = case shown="\"other\", Default" w68 {
          tunnel: [Sample_Type."Empty Resonator" ("Sample Type") Sample_Type."LiPc" ("Sample Type") Sample_Type."OxyChip" ("Sample Type") Sample_Type."India Ink" ("Sample Type")] -> w70
          frame "other", Default {
          }
          frame "lipc" {
          }
          frame "oxychip" {
          }
          frame "carloerba" {
          }
        }
      }
    }
    n43 = To Lower Case(string=w19) -> (all lower case string=w28:string)
    n44 = Equal?(x="other", y=w28) -> (x = y?=w25:bool)
    n45 = property on="Manual Sample Input" class="Str"("Visible"=w25) -> ()  [unwired: 2 in, 2 out]
    n46 = Select(t="Manual Sample Input", s=w25, f=w18) -> (s? t:f=w26:string)
  }
  "Resonator ID" <- w13
  "Sample Selected" <- w12
  "Gases Used" <- w11
  "Fraction O2" <- w10
  "Sample Type" <- w1
